vi "Laser MARKED V1.vi"(8 "error in":errorcluster, 9 "LaserOffSet":string, 10 "Sn":string, 11 "Marked Type":string="bf1-1") -> (0 "error constant":errorcluster)   [LabVIEW 2019]
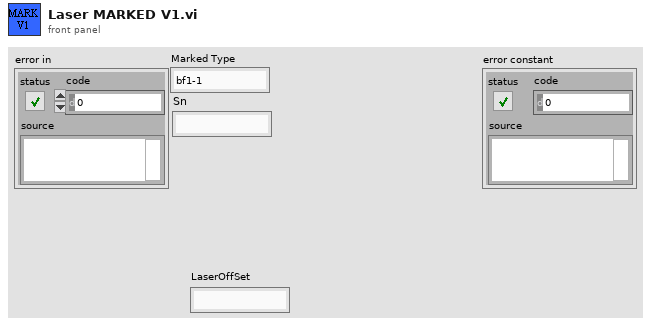
[diagram p1: front panel]
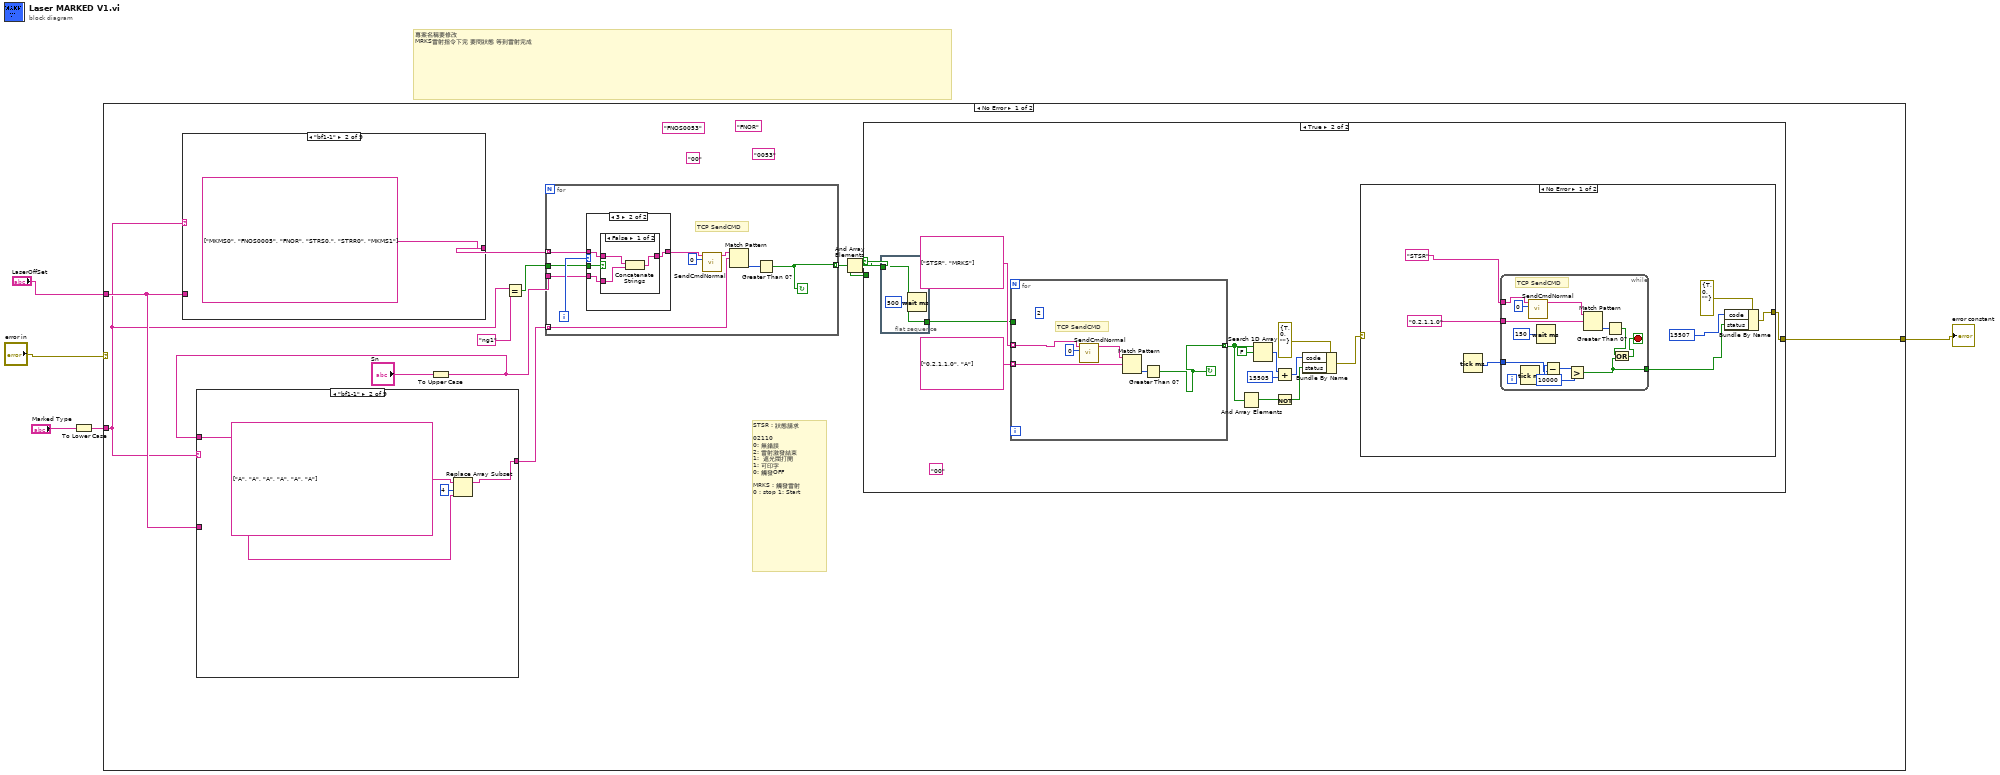
[diagram p0: block diagram]
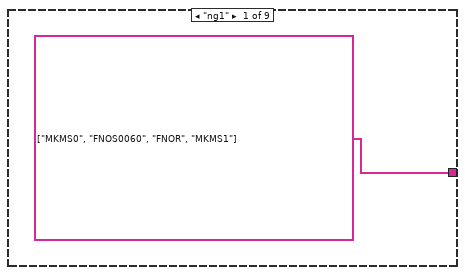
[diagram p2: hidden frame]
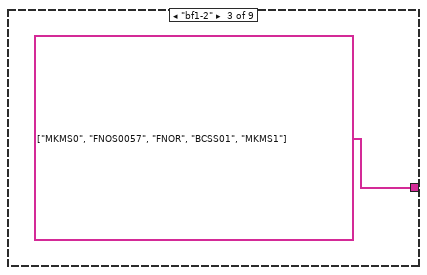
[diagram p3: hidden frame]
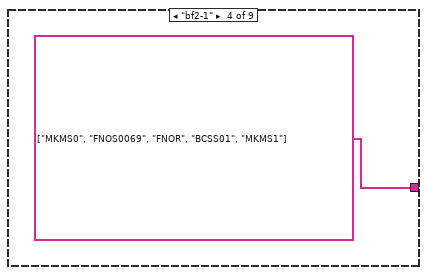
[diagram p4: hidden frame]
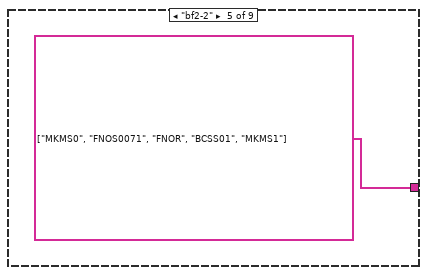
[diagram p5: hidden frame]
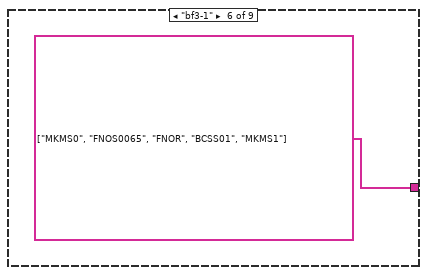
[diagram p6: hidden frame]
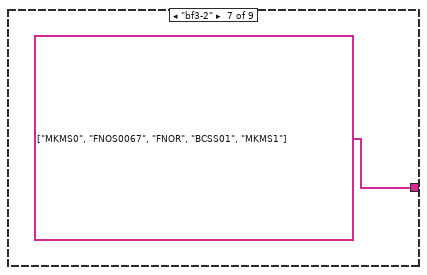
[diagram p7: hidden frame]
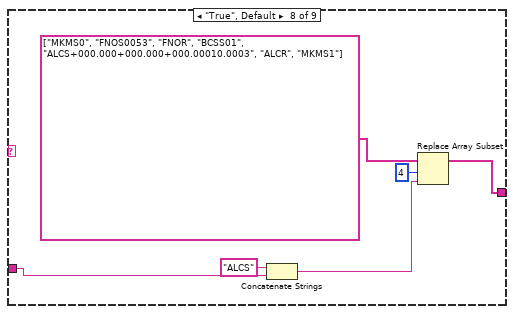
[diagram p8: hidden frame]
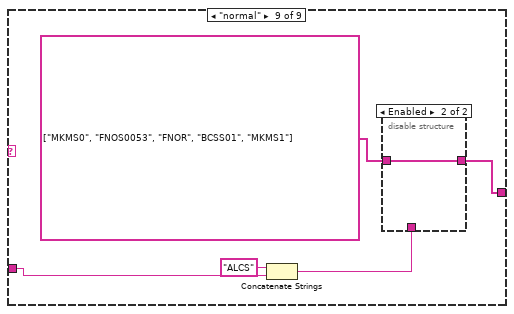
[diagram p9: hidden frame]
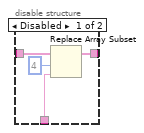
[diagram p10: hidden frame]
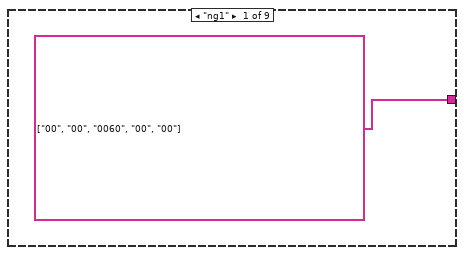
[diagram p11: hidden frame]
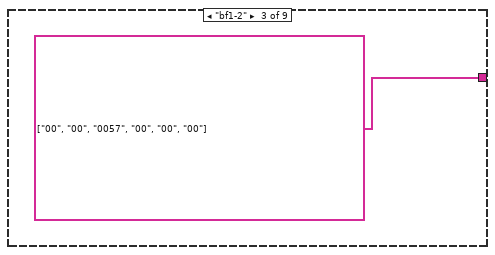
[diagram p12: hidden frame]
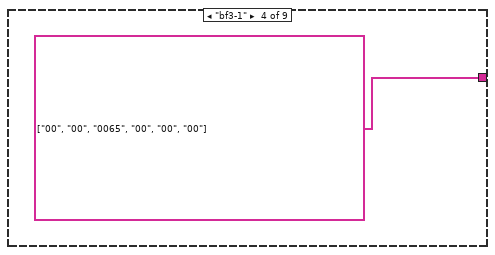
[diagram p13: hidden frame]
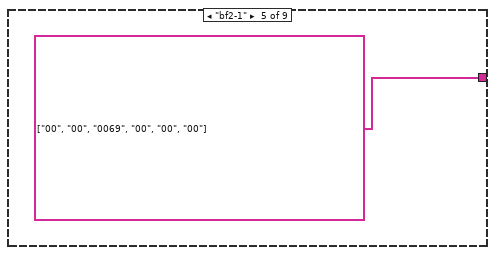
[diagram p14: hidden frame]
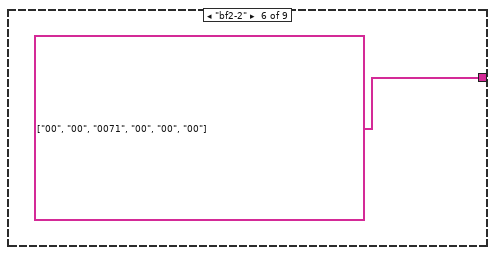
[diagram p15: hidden frame]
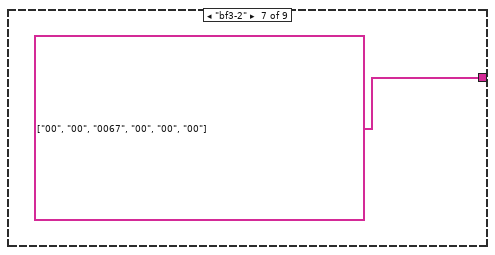
[diagram p16: hidden frame]
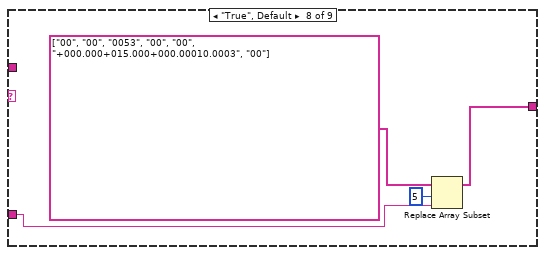
[diagram p17: hidden frame]
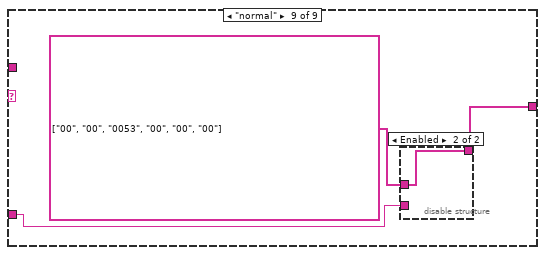
[diagram p18: hidden frame]
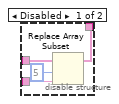
[diagram p19: hidden frame]
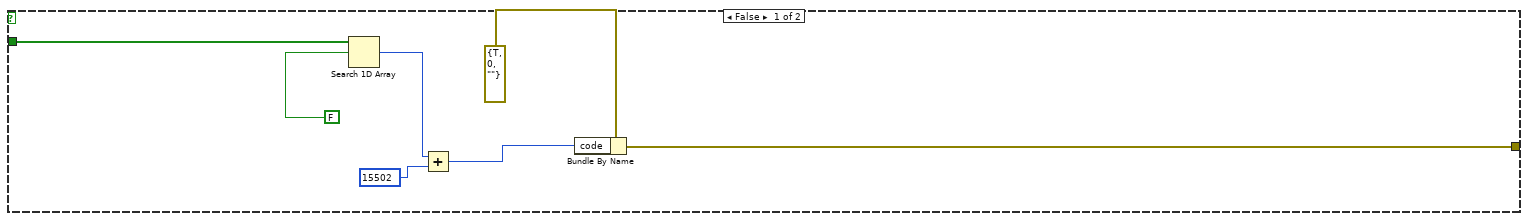
[diagram p20: hidden frame]
diagram:
  # "專案名稱要修改\nMRKS雷射指令下完 要問狀態 等到雷射完成"
  n1 = To Lower Case(string="Marked Type") -> (all lower case string=w1:string)
  n2 = case shown="No Error" "error in" {
    selector: "error in" -> [_ w131]
    tunnel: [w12 w131] -> w4
    tunnel: w1 -> [w9 _]
    tunnel: "LaserOffSet" -> [w11 _]
    frame No Error {
      (unwired) "0053" ("String")
      (unwired) "FNOR" ("String")
      (unwired) "00" ("String")
      (unwired) "FNOS0053" ("String")
      # "STSR : 狀態請求\n\n02110\n0: 無錯誤\n2: 雷射激發結束\n1:  遮光閥打開\n1: 可印字\n0: 觸發OFF\n\nMRKS : 觸發雷射 \n0 : stop 1: Start"
      n3 = case shown="\"bf1-1\"" w9 {
        tunnel: [string[] ["MKMS0", "FNOS0060", "FNOR", "MKMS1"] ("Array") string[] ["MKMS0", "FNOS0005", "FNOR", "STRS0,", "STRR0", "MKMS1"] ("Array") string[] ["MKMS0", "FNOS0057", "FNOR", "BCSS01", "MKMS1"] ("Array") string[] ["MKMS0", "FNOS0069", "FNOR", "BCSS01", "MKMS1"] ("Array") string[] ["MKMS0", "FNOS0071", "FNOR", "BCSS01", "MKMS1"] ("Array") string[] ["MKMS0", "FNOS0065", "FNOR", "BCSS01", "MKMS1"] ("Array") string[] ["MKMS0", "FNOS0067", "FNOR", "BCSS01", "MKMS1"] ("Array") w27 w33] -> w16
        tunnel: w11 -> [_ _ _ _ _ _ _ w26 w32]
        frame "ng1" {
        }
        frame "bf1-1" {
        }
        frame "bf1-2" {
        }
        frame "bf2-1" {
        }
        frame "bf2-2" {
        }
        frame "bf3-1" {
        }
        frame "bf3-2" {
        }
        frame "True", Default {
          n4 = Concatenate Strings("ALCS" ("string"), w26) -> (w24:string)
          n5 = Replace Array Subset(array=string[] ["MKMS0", "FNOS0053", "FNOR", "BCSS01", "ALCS+000.000+000.000+000.00010.0003", "ALCR", "MKMS1"] ("Array"), new element=w24, index=4) -> (w27:string[])
        }
        frame "normal" {
          n6 = Concatenate Strings("ALCS" ("string"), w32) -> (w30:string)
          n7 = disable-structure shown="Enabled" {
            disable-tunnel: string[] ["MKMS0", "FNOS0053", "FNOR", "BCSS01", "MKMS1"] ("Array") -> [w38 w39]
            disable-tunnel: [w36 w39] -> w33
            disable-tunnel: w30 -> [w35 _]
            frame Disabled {
              n8 = Replace Array Subset(array=w38, new element=w35, index=4) -> (w36:string[])
            }
            frame Enabled {
            }
          }
        }
      }
      n9 = To Upper Case(1:"Sn") -> (0:w6:string)
      n10 = case shown="\"bf1-1\"" w9 {
        tunnel: [string[] ["00", "00", "0060", "00", "00"] ("Array") w43 string[] ["00", "00", "0057", "00", "00", "00"] ("Array") string[] ["00", "00", "0065", "00", "00", "00"] ("Array") string[] ["00", "00", "0069", "00", "00", "00"] ("Array") string[] ["00", "00", "0071", "00", "00", "00"] ("Array") string[] ["00", "00", "0067", "00", "00", "00"] ("Array") w50 w54] -> w13
        tunnel: w11 -> [_ _ _ _ _ _ _ w52 w55]
        tunnel: w6 -> [_ w41 _ _ _ _ _ _ _]
        frame "ng1" {
        }
        frame "bf1-1" {
          n11 = Replace Array Subset(array=string[] ["A", "A", "A", "A", "A", "A"] ("Array"), new element=w41, index=4) -> (w43:string[])
        }
        frame "bf1-2" {
        }
        frame "bf3-1" {
        }
        frame "bf2-1" {
        }
        frame "bf2-2" {
        }
        frame "bf3-2" {
        }
        frame "True", Default {
          n12 = Replace Array Subset(array=string[] ["00", "00", "0053", "00", "00", "+000.000+015.000+000.00010.0003", "00"] ("Array"), new element=w52, index=5) -> (w50:string[])
        }
        frame "normal" {
          n13 = disable-structure shown="Enabled" {
            disable-tunnel: string[] ["00", "00", "0053", "00", "00", "00"] ("Array") -> [w60 w61]
            disable-tunnel: w55 -> [w59 _]
            disable-tunnel: [w57 w61] -> w54
            frame Disabled {
              n14 = Replace Array Subset(array=w60, new element=w59, index=5) -> (w57:string[])
            }
            frame Enabled {
            }
          }
        }
      }
      n15 = Equal?(x=w9, y="ng1") -> (x = y?=w10:bool)
      n16 = for {
        tunnel: w16 -> [w119] mode=indexing
        tunnel: w6 -> [w118]
        tunnel: [w117] -> w14 mode=indexing
        tunnel: w13 -> [w116] mode=indexing
        tunnel: w10 -> [w115]
        i -> [w120]
        stop <- w117 continue-if-true
        # "TCP SendCMD"
        n17 = case shown="3" w120 {
          tunnel: w119 -> [w122 w126]
          tunnel: [w122 w125] -> w113
          tunnel: w118 -> [_ w124]
          tunnel: w115 -> [_ w123]
          frame 0, Default {
          }
          frame 3 {
            n18 = case shown="False" w123 {
              tunnel: w126 -> [w129 w130]
              tunnel: [w128 w130] -> w125
              tunnel: w124 -> [w127 _]
              frame False {
                n19 = Concatenate Strings(w129, w127) -> (w128:string)
              }
              frame True {
              }
            }
          }
        }
        n20 = call "SendCmdNormal.vi"("index"=0, "DataIn"=w113) -> ("Reccmd"=w114:string)  [unwired: 7 in, 2 out]
        n21 = Match Pattern(string=w114, regular expression=w116) -> (offset past match=w121:i32)  [unwired: 1 in, 3 out]
        n22 = Greater Than 0?(x=w121) -> (x > 0?=w117:bool)
      }
      n23 = And Array Elements(Boolean array=w14) -> (logical AND=w15:bool)
      n24 = case shown="True" w15 {
        selector: w15 -> [_ w70]
        tunnel: w14 -> [w68 _]
        tunnel: [w62 w71] -> w12
        frame False {
          n25 = Search 1D Array(1D array=w68, element=FALSE) -> (index of element=w66:i32)  [unwired: 1 in]
          n26 = Add(x=w66, y=15502) -> (x+y=w63:i32)
          n27 = Bundle By Name(cluster=errorcluster {"status"=TRUE, "code"=0, "source"=""} ("error constant"), "code"=w63) -> (w62:errorcluster)
        }
        frame True {
          (unwired) "00"
          n28 = flat-sequence {
            tunnel: w70 -> [w83]
            tunnel: [w83] -> w69
            frame #0 {
              n29 = Wait (ms)(milliseconds to wait=u32 500) -> ()  [unwired: 1 out]
            }
          }
          n30 = for {
            tunnel: string[] ["STSR", "MRKS"] ("Array") -> [w106] mode=indexing
            tunnel: [w109] -> w78 mode=indexing
            tunnel: string[] ["0,2,1,1,0", "A"] ("Array") -> [w111] mode=indexing
            tunnel: w69 -> [_]
            stop <- w109 continue-if-true
            (unwired) 2
            # "TCP SendCMD"
            n31 = call "SendCmdNormal.vi"("index"=0, "DataIn"=w106) -> ("Reccmd"=w107:string)  [unwired: 7 in, 2 out]
            n32 = Match Pattern(string=w107, regular expression=w111) -> (offset past match=w110:i32)  [unwired: 1 in, 3 out]
            n33 = Greater Than 0?(x=w110) -> (x > 0?=w109:bool)
          }
          n34 = And Array Elements(Boolean array=w78) -> (logical AND=w77:bool)
          n35 = Search 1D Array(1D array=w78, element=FALSE) -> (index of element=w81:i32)  [unwired: 1 in]
          n36 = Add(x=w81, y=15505) -> (x+y=w79:i32)
          n37 = Not(x=w77) -> (.not. x?=w75:bool)
          n38 = Bundle By Name(cluster=errorcluster {"status"=TRUE, "code"=0, "source"=""} ("error constant"), "code"=w79, "status"=w75) -> (w72:errorcluster)
          n39 = case shown="No Error" w72 {
            selector: w72 -> [_ w105]
            tunnel: [w87 w105] -> w71
            frame No Error {
              n40 = Tick Count (ms)() -> (millisecond timer value=w89:u32)
              n41 = while {
                tunnel: "STSR" ("String") -> [w92]
                tunnel: "0,2,1,1,0" ("String") -> [w102]
                tunnel: w89 -> [w100]
                tunnel: [w95] -> w91
                stop <- w96 stop-if-true
                # "TCP SendCMD"
                n42 = Tick Count (ms)() -> (millisecond timer value=w101:u32)
                n43 = call "SendCmdNormal.vi"("index"=0, "DataIn"=w92) -> ("Reccmd"=w93:string)  [unwired: 7 in, 2 out]
                n44 = Wait (ms)(milliseconds to wait=u32 150 ("millisecond timer value")) -> ()  [unwired: 1 out]
                n45 = Subtract(x=w101, y=w100) -> (x-y=w99:u32)
                n46 = Greater?(x=w99, y=u32 10000) -> (0:w95:bool)
                n47 = Match Pattern(string=w93, regular expression=w102) -> (offset past match=w103:i32)  [unwired: 1 in, 3 out]
                n48 = Greater Than 0?(x=w103) -> (x > 0?=w97:bool)
                n49 = Or(x=w97, y=w95) -> (x .or. y?=w96:bool)
              }
              n50 = Bundle By Name(cluster=errorcluster {"status"=TRUE, "code"=0, "source"=""} ("error constant"), "code"=15507, "status"=w91) -> (w87:errorcluster)
            }
            frame Error {
            }
          }
        }
      }
    }
    frame Error {
    }
  }
  "error constant" <- w4
